vi "Read Modulation.vi"(8 "error in (no error)":errorcluster, 11 "Set Modulation MSG in":refnum<class "Set Modulation MSG.lvclass">) -> (0 "error out":errorcluster, 2 "Modulation":enum8{"Sine", "Square"}[](array[ring]), 3 "Set Modulation MSG out":refnum<class "Set Modulation MSG.lvclass">)   [LabVIEW 2014, in "ePAS Library.lvlib" / "Set Modulation MSG.lvclass"]
uses:
  Set Modulation MSG.lvclass
  Set Modulation MSG.lvclass/Set Modulation MSG.ctl
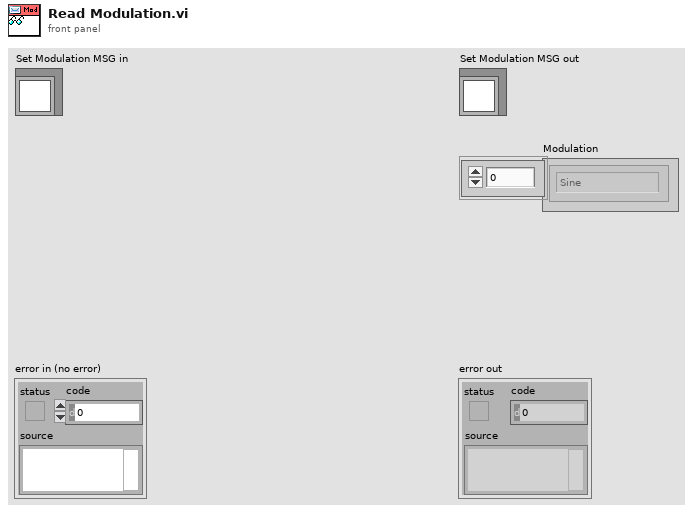
[diagram p1: front panel]
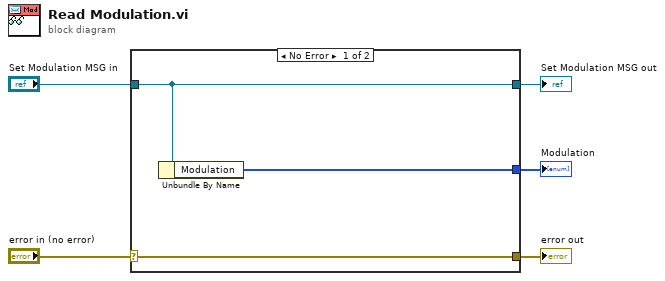
[diagram p0: block diagram]
diagram:
  n1 = case shown="No Error" "error in (no error)" {
    selector: "error in (no error)" -> [w8 w9]
    tunnel: [w8 w9] -> w4
    tunnel: [w7 w10] -> w2
    tunnel: "Set Modulation MSG in" -> [w7 w10]
    tunnel: [w6 _] -> w1
    frame No Error {
      n2 = Unbundle By Name(w7) -> ("Modulation"=w6:enum8{"Sine", "Square"}[])
    }
    frame Error {
    }
  }
  "error out" <- w4
  "Set Modulation MSG out" <- w2
  "Modulation" <- w1
